vi "Write File.vi"(8 "error in (no error)":errorcluster, 11 "[User] Cfg File in":refnum<class "[User] Cfg File.lvclass">) -> (0 "error out":errorcluster, 3 "[User] Cfg File out":refnum<class "[User] Cfg File.lvclass">)   [LabVIEW 2020, in "[User] Cfg File.lvclass"]
uses:
  [User] Cfg File.lvclass
  [User] Cfg File.lvclass/[User] Cfg File.ctl
  <vilib>/Utility/config.llb/NI_LVConfig.lvlib
  <userlib>/_OpenG.lib/variantconfig/variantconfig.llb/openg_variant_configuration_file.lvlib
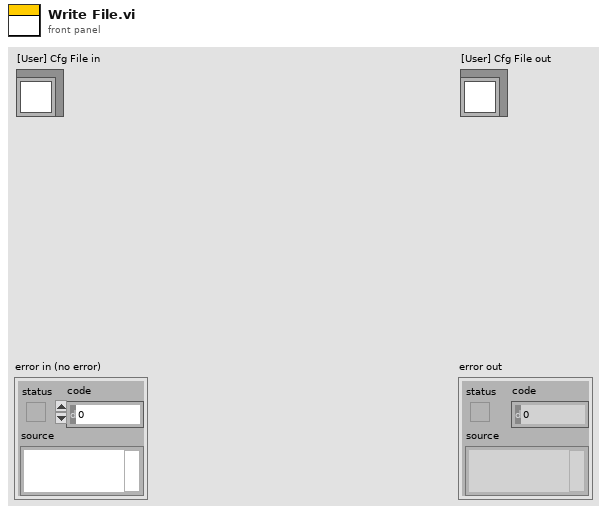
[diagram p1: front panel]
types:
  T1 = typedef "NI_LVConfig.lvlib/Config Data RefNum.ctl" = refnum<k1>
  T2 = typedef "[User] Cfg File.lvclass/config file.ctl" = cluster{"login":cluster{"rmb_user":bool}}
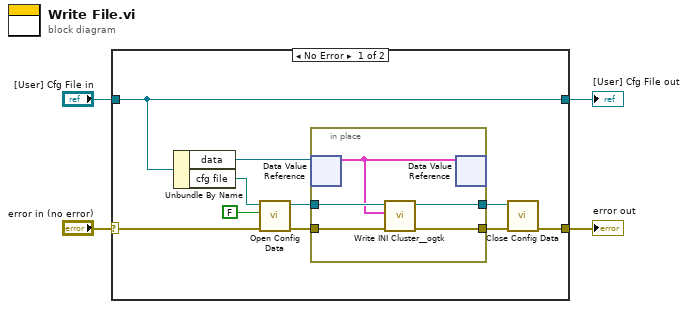
[diagram p0: block diagram]
diagram:
  n1 = case shown="No Error" "error in (no error)" {
    selector: "error in (no error)" -> [w12 w21]
    tunnel: [w5 w21] -> w3
    tunnel: [w14 w20] -> w1
    tunnel: "[User] Cfg File in" -> [w14 w20]
    frame No Error {
      n2 = Unbundle By Name(w14) -> ("data"=w13:refnum<data-value>, "cfg file"=w11:path)
      n3 = call <vilib>:"Open Config Data.vi"("error in (no error)"=w12, "create file if necessary (T)"=FALSE, "configuration file path"=w11) -> ("error out"=w8:errorcluster, "refnum"=w9:T1)  [unwired: 6 in, 1 out]
      n4 = in-place {
        in-place-border: w9 -> [w18]
        in-place-border: w8 -> [w19]
        in-place-border: [w16] -> w6
        in-place-border: [w15] -> w7
        n5 = in-place-dvr #1(w13) -> (w17:T2)  [unwired: 1 out]
        n6 = call <userlib>:"Write INI Cluster__ogtk.vi"("error in (no error)"=w19, "INI Fomatted Cluster"=w17, "refnum"=w18) -> ("error out"=w15:errorcluster, "dup refnum"=w16:T1)  [unwired: 7 in]
        n7 = in-place-dvr #1(w17) -> ()  [unwired: 2 out]
      }
      n8 = call <vilib>:"Close Config Data.vi"("error in (no error)"=w7, "refnum"=w6) -> ("error out"=w5:errorcluster)  [unwired: 8 in, 1 out]
    }
    frame Error {
    }
  }
  "error out" <- w3
  "[User] Cfg File out" <- w1
